vi "h5_2D_I16.vi"(6 "Attributes":variant, 7 "TYPE":string="CAM", 8 "error in (no error)":errorcluster, 9 "2D I16":i16[][](array[numeric]), 10 "SQUID":string, 11 "H5":path[](array[path])) -> (0 "error out":errorcluster, 1 "Repeat":i32, 2 "Exists":bool)   [LabVIEW 2013]
uses:
  <vilib>/addons/h5labview2/file/H5Fmode.ctl
  <vilib>/addons/h5labview2/base/lib_path.vi
  <vilib>/addons/h5labview2/base/H5Equery.vi
  <vilib>/addons/h5labview2/base/hid_t.ctl
  <vilib>/addons/h5labview2/dataset/H5Dwrite.llb/H5Dwrite.xnode
  <vilib>/addons/h5labview2/file/H5F.lvlib
  <vilib>/addons/h5labview2/group/H5G.lvlib
  <vilib>/addons/h5labview2/attrib/H5A.lvlib
panel:
  out "error out 2":errorcluster
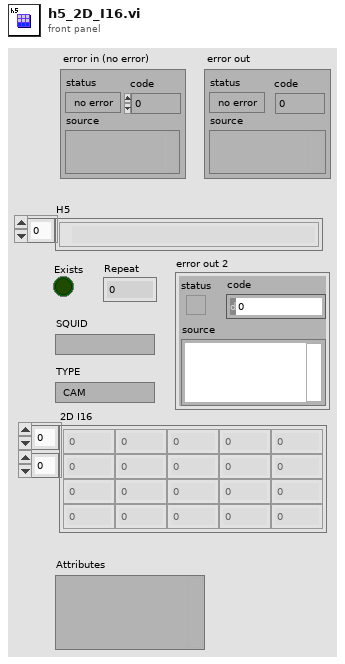
[diagram p1: front panel]
types:
  T1 = typedef "Semaphore RefNum" = refnum<k1>
  T2 = typedef "H5F.lvlib/H5Fmode.ctl" = enum16{"read-only", "read-write", "overwrite", "create new", "open or create"}
  T3 = typedef "hid_t.ctl" = i32
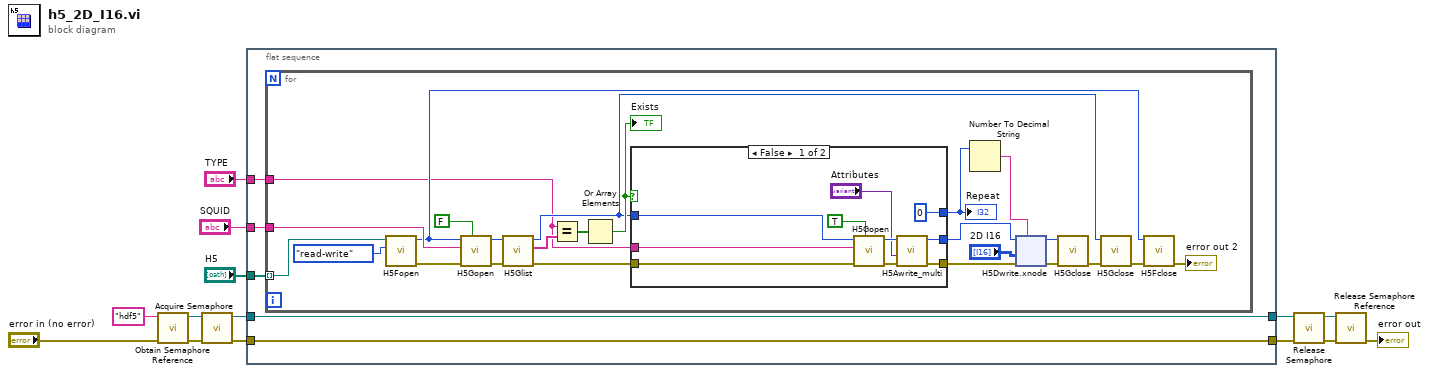
[diagram p0: block diagram]
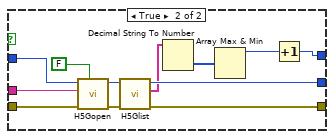
[diagram p2: hidden frame]
diagram:
  n1 = call <vilib>:"Obtain Semaphore Reference.vi"("error in (no error)"="error in (no error)", "name (unnamed)"="hdf5") -> ("error out"=w13:errorcluster, "semaphore"=w14:T1)  [unwired: 3 in, 1 out]
  n2 = call <vilib>:"Acquire Semaphore.vi"("error in (no error)"=w13, "semaphore"=w14) -> ("error out"=w7:errorcluster, "semaphore out"=w6:T1)  [unwired: 3 in, 1 out]
  n3 = flat-sequence {
    tunnel: [w19] -> w8
    tunnel: w7 -> [w19]
    tunnel: w6 -> [w18]
    tunnel: [w18] -> w5
    tunnel: "H5" -> [w17]
    tunnel: "SQUID" -> [w16]
    tunnel: "TYPE" -> [w15]
    frame #0 {
      n4 = for {
        tunnel: w17 -> [w38] mode=indexing
        tunnel: w16 -> [w39]
        tunnel: w15 -> [w29]
        n5 = call <vilib>:"H5Fopen.vi"("mode (read-only)"=H5Fmode."read-write", "path"=w38) -> ("error out"=w37:errorcluster, "ref out"=w36:T3)  [unwired: 8 in]
        n6 = call <vilib>:"H5Gopen.vi"("create? (F)"=FALSE, "error in (no error)"=w37, "name"=w39, "ref in"=w36) -> ("error out"=w34:errorcluster, "group out"=w35:T3)  [unwired: 6 in]
        n7 = call <vilib>:"H5Glist.vi"("error in (no error)"=w34, "ref in"=w35) -> ("error out"=w28:errorcluster, "names"=w33:string[], "ref out"=w30:T3)  [unwired: 6 in, 1 out]
        n8 = Equal?(x=w29, y=w33) -> (x = y?=w32:bool[])
        n9 = Or Array Elements(Boolean array=w32) -> (logical OR=w31:bool)
        "Exists" <- w31
        n10 = case shown="False" w31 {
          tunnel: w30 -> [w52 w62]
          tunnel: w29 -> [w51 w63]
          tunnel: w28 -> [w50 w64]
          tunnel: [w47 w60] -> w25
          tunnel: [w46 w58] -> w26
          tunnel: [0 w54] -> w20
          frame False {
            n11 = call <vilib>:"H5Gopen.vi"("create? (F)"=TRUE, "error in (no error)"=w50, "name"=w51, "ref in"=w52) -> ("error out"=w48:errorcluster, "group out"=w45:T3)  [unwired: 6 in]
            n12 = call <vilib>:"H5Awrite_multi.vi"("error in (no error)"=w48, "variant in"="Attributes", "ref in"=w45) -> ("error out"=w47:errorcluster, "ref out"=w46:T3)  [unwired: 7 in]
          }
          frame True {
            n13 = call <vilib>:"H5Gopen.vi"("create? (F)"=FALSE, "error in (no error)"=w64, "name"=w63, "ref in"=w62) -> ("error out"=w61:errorcluster, "group out"=w59:T3)  [unwired: 6 in]
            n14 = call <vilib>:"H5Glist.vi"("error in (no error)"=w61, "ref in"=w59) -> ("error out"=w60:errorcluster, "names"=w57:string[], "ref out"=w58:T3)  [unwired: 6 in, 1 out]
            n15 = Decimal String To Number(string=w57) -> (number=w56:i32[])  [unwired: 2 in, 1 out]
            n16 = Array Max & Min(array=w56) -> (max value=w55:i32)  [unwired: 3 out]
            n17 = Increment(x=w55) -> (x+1=w54:i32)
          }
        }
        "Repeat" <- w20
        n18 = Number To Decimal String(number=w20) -> (decimal integer string=w21:string)  [unwired: 1 in]
        n19 = xnode "H5Dwrite.xnode"("dataset name"=w21, "error in (no error)"=w25, "data"="2D I16", "ref in"=w26) -> ("error out"=w23:errorcluster, "ref out"=w24:T3)  [unwired: 3 in, 1 out]
        n20 = call <vilib>:"H5Gclose.vi"("error in (no error)"=w23, "group in"=w24) -> ("error out"=w22:errorcluster)  [unwired: 9 in]
        n21 = call <vilib>:"H5Gclose.vi"("error in (no error)"=w22, "group in"=w30) -> ("error out"=w40:errorcluster)  [unwired: 9 in]
        n22 = call <vilib>:"H5Fclose.vi"("error in (no error)"=w40, "ref"=w36) -> ("error out"=→"error out 2":errorcluster)  [unwired: 9 in]
      }
    }
  }
  n23 = call <vilib>:"Release Semaphore.vi"("error in (no error)"=w8, "semaphore"=w5) -> ("error out"=w9:errorcluster, "semaphore out"=w10:T1)  [unwired: 4 in]
  n24 = call <vilib>:"Release Semaphore Reference.vi"("error in (no error)"=w9, "semaphore"=w10) -> ("error out"=→"error out":errorcluster)  [unwired: 8 in, 1 out]
